vi "GetTemplatePath.vi"(0 "reference in":refnum<class "ClassWriterGOOP400.lvclass">, 1 "ClassTemplateSubDirectory":string, 5 "error in (no error)":errorcluster) -> (14 "reference out":refnum<class "ClassWriterGOOP400.lvclass">, 15 "FolderPathOut":path, 17 "MethodTemplatePathOut":path, 18 "TemplateSettings":T1, 19 "error out":errorcluster)   [LabVIEW 2016, in "ClassWriterGOOP400.lvclass"]
uses:
  <resource>/Framework/Providers/Open_GDS/ClassProviders/Provider_EndevoGOOP400/ClassWriterGOOP400_class/ClassWriterGOOP400.lvclass
  <resource>/Framework/Providers/Open_GDS/ClassProviders/Provider_BaseClassInterface/ClassWriter_class/TemplateSettings.ctl
  <resource>/Framework/Providers/Open_GDS/ClassProviders/Provider_LvNativeClass/ClassWriterNative_class/ClassWriterNative.lvclass
  <resource>/Framework/Providers/Open_GDS/ClassProviders/Provider_BaseClassInterface/ClassWriter_class/ClassWriter.lvclass
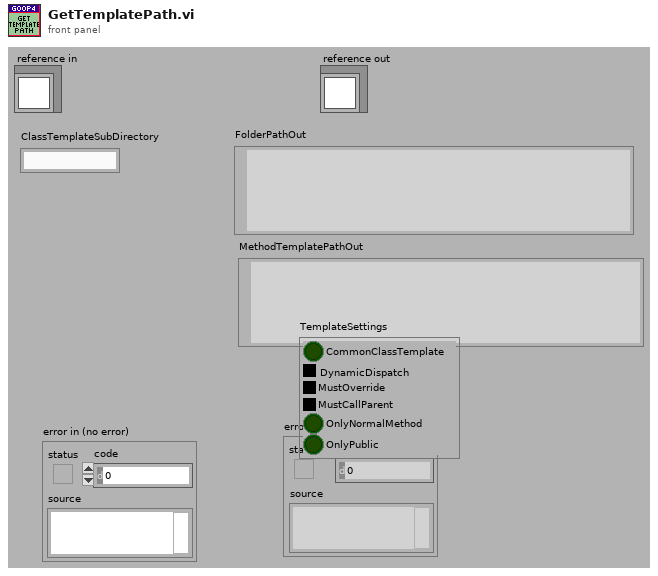
[diagram p1: front panel]
types:
  T1 = typedef "ClassWriter.lvclass/TemplateSettings.ctl" = cluster{"CommonClassTemplate":bool, "DynamicDispatch":enum8{"False", "True", "Mixed"}, "MustOverride":enum8{"False", "True", "Mixed"}, "MustCallParent":enum8{"False", "True", "Mixed"}, "OnlyNormalMethod":bool, "OnlyPublic":bool}
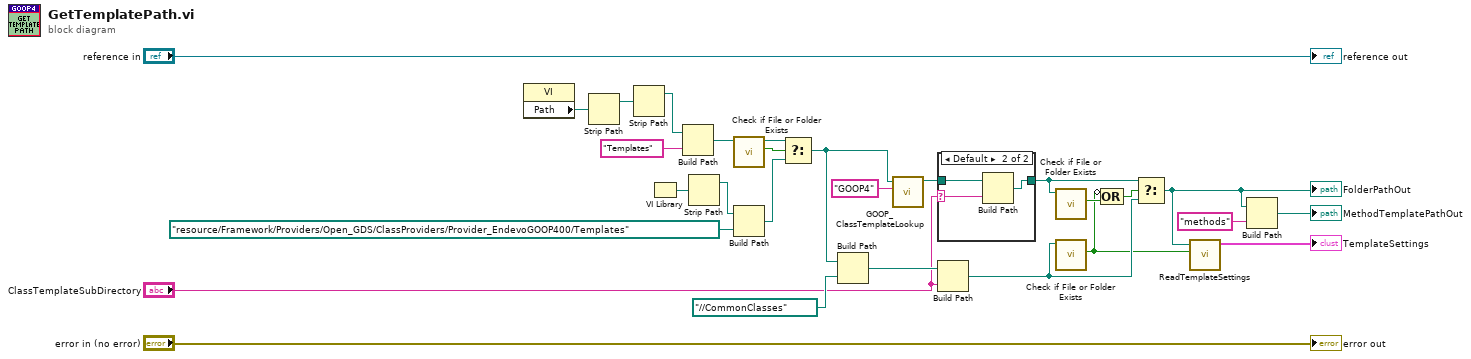
[diagram p0: block diagram]
diagram:
  n1 = property class="VI"() -> ("Path"=w26:path)  [unwired: 2 in, 2 out]
  n2 = Strip Path(path=w26) -> (stripped path=w24:path)  [unwired: 1 out]
  n3 = Strip Path(path=w24) -> (stripped path=w28:path)  [unwired: 1 out]
  n4 = VI Library() -> (path=w20:path)
  n5 = Build Path(base path=w28, name or relative path="Templates") -> (appended path=w21:path)
  n6 = Strip Path(path=w20) -> (stripped path=w14:path)  [unwired: 1 out]
  n7 = call <vilib>:"Check if File or Folder Exists.vi"("path"=w21) -> ("file or folder exists?"=w23:bool, "dup path"=w22:path)  [unwired: 8 in, 1 out]
  n8 = Build Path(base path=w14, name or relative path=path "resource/Framework/Providers/Open_GDS/ClassProviders/Provider_EndevoGOOP400/Templates" ("base path")) -> (appended path=w18:path)
  n9 = Select(t=w22, s=w23, f=w18) -> (s? t:f=w7:path)
  n10 = Build Path(base path=w7, name or relative path=path "../../CommonClasses") -> (appended path=w10:path)
  n11 = call <resource>:"GOOP_ClassTemplateLookup.vi"("ClassType"="GOOP4", "ClassTemplateFolderIn"=w7) -> ("ClassTemplateFolderOut"=w12:path)  [unwired: 9 in]
  n12 = case shown="Default" "ClassTemplateSubDirectory" {
    selector: "ClassTemplateSubDirectory" -> [_ w30]
    tunnel: w12 -> [w29 w32]
    tunnel: [w29 w31] -> w8
    frame "" {
    }
    frame Default {
      n13 = Build Path(base path=w32, name or relative path=w30) -> (appended path=w31:path)
    }
  }
  n14 = Build Path(base path=w10, name or relative path="ClassTemplateSubDirectory") -> (appended path=w4:path)
  n15 = call <vilib>:"Check if File or Folder Exists.vi"("path"=w8) -> ("file or folder exists?"=w3:bool)  [unwired: 8 in, 2 out]
  n16 = call <vilib>:"Check if File or Folder Exists.vi"("path"=w4) -> ("file or folder exists?"=w1:bool)  [unwired: 8 in, 2 out]
  n17 = Compound Arithmetic op=OR(invert w1, w3) -> (w2:bool)
  n18 = Select(t=w8, s=w2, f=w4) -> (s? t:f=w5:path)
  "FolderPathOut" <- w5
  n19 = call <resource>:"ReadTemplateSettings.vi"("CommonClassTemplate"=w1, "TemplateFolder"=w5) -> ("TemplateSettings"=→"TemplateSettings":T1)  [unwired: 9 in]
  n20 = Build Path(base path=w5, name or relative path="methods") -> (appended path=→"MethodTemplatePathOut":path)
  "error out" <- "error in (no error)"
  "reference out" <- "reference in"
